vi "Log Data_RT.vi"(5 "FPGA VI Reference":T1, 7 "Total Buffer Size":i32, 8 "error in (no error)":errorcluster, 10 "Acquisition and Logging Configuration":T2={"Data Rate"=1, "Samples per Read"=0, "Number of Reads to Save"=0, "Data File Name"="", "TDMS Properties"=[], "Number of Channels"=4, "Channel Scale Array"=[0.0, 0.0, 0.0, 0.0, 1.0, 1.0, 1.0, 1.0], "Channel Names"=[], "Trigger - RMS Value"=0.0, "Trigger - Channel"=0, "Trigger - Time (Minute)"=0} {"Data Rate" items=["51.200 kS/s (NI 9234)"=1, "25.600 kS/s (NI 9234)"=2, "17.067 kS/s (NI 9234)"=3, "12.800 kS/s (NI 9234)"=4, "10.240 kS/s (NI 9234)"=5, "8.533 kS/s (NI 9234)"=6, "7.314 kS/s (NI 9234)"=7, "6.400 kS/s (NI 9234)"=8, "5.689 kS/s (NI 9234)"=9, "5.120 kS/s (NI 9234)"=10, "4.654 kS/s (NI 9234)"=11, "4.267 kS/s (NI 9234)"=12, "3.938 kS/s (NI 9234)"=13, "3.657 kS/s (NI 9234)"=14, "3.413 kS/s (NI 9234)"=15, "3.200 kS/s (NI 9234)"=16, "3.012 kS/s (NI 9234)"=17, "2.845 kS/s (NI 9234)"=18, "2.695 kS/s (NI 9234)"=19, "2.560 kS/s (NI 9234)"=20, "2.438 kS/s (NI 9234)"=21, "2.328 kS/s (NI 9234)"=22, "2.226 kS/s (NI 9234)"=23, "2.133 kS/s (NI 9234)"=24, "2.048 kS/s (NI 9234)"=25, "1.969 kS/s (NI 9234)"=26, "1.896 kS/s (NI 9234)"=27, "1.829 kS/s (NI 9234)"=28, "1.765 kS/s (NI 9234)"=29, "1.707 kS/s (NI 9234)"=30, "1.652 kS/s (NI 9234)"=31]}, 11 "rt fifo":refnum<k33>) -> (0 "error out":errorcluster)   [LabVIEW 2015]
doc: "Reads waveform data from the DMA FIFO."
uses:
  Globals/Global - Monitoring Variables.vi
  <vilib>/LabVIEW Targets/FPGA/cRIO/shared/nicrio_ModuleControls/nicrio_cRIO-9234_DataRatesRing2.ctl
  controls/Acquisition and Logging Configuration.ctl
  controls/FPGA VI Reference.ctl
  controls/TDMS Properties.ctl
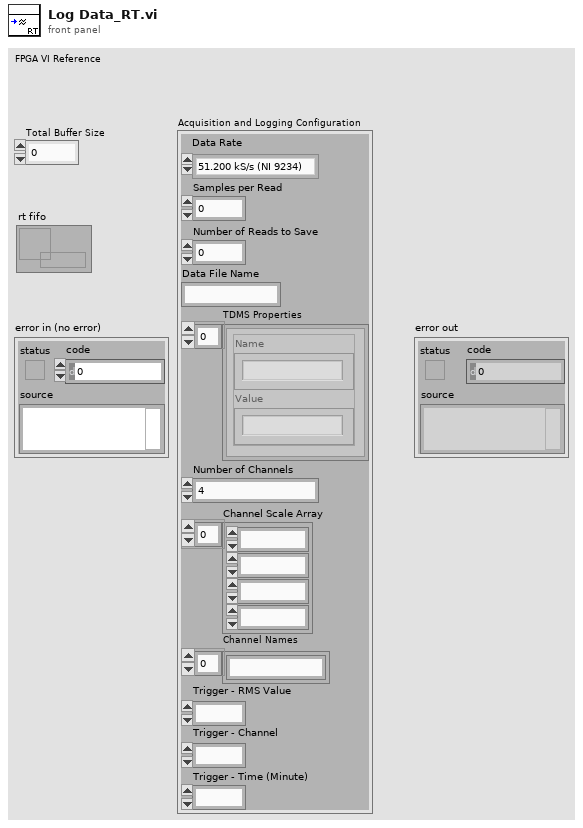
[diagram p1: front panel]
types:
  T1 = typedef "FPGA VI Reference.ctl" = refnum<k20>
  T2 = typedef "Acquisition and Logging Configuration.ctl" = cluster{"Data Rate":T3, "Samples per Read":i32, "Number of Reads to Save":i32, "Data File Name":string, "TDMS Properties":T4[], "Number of Channels":i32, "Channel Scale Array":fxp<+,24,12>[], "Channel Names":string[], "Trigger - RMS Value":dbl, "Trigger - Channel":i32, "Trigger - Time (Minute)":i32}
  T3 = typedef "nicrio_cRIO-9234_DataRatesRing2.ctl" = u8
  T4 = typedef "TDMS Properties.ctl" = cluster{"Name":string, "Value":string}
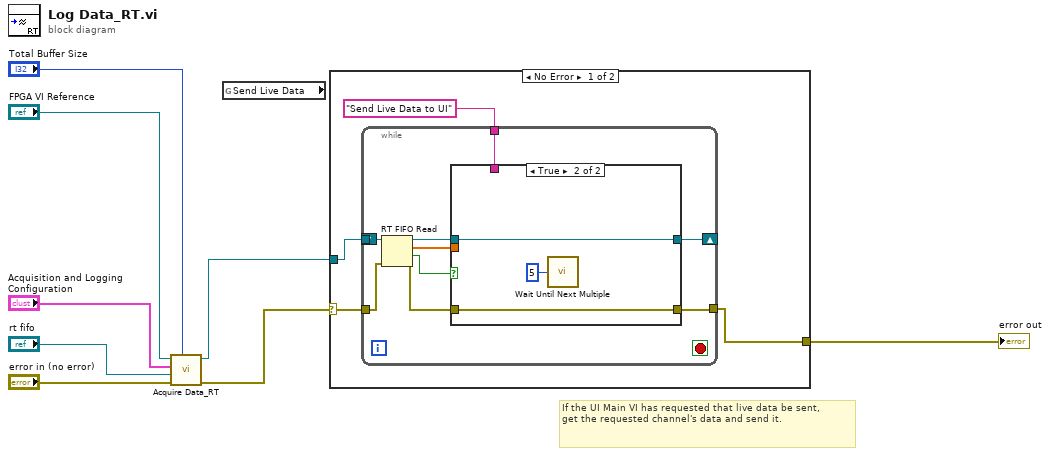
[diagram p0: block diagram]
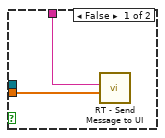
[diagram p2: hidden frame]
diagram:
  # "If the UI Main VI has requested that live data be sent,\nget the requested channel's data and send it."
  n1 = call "Acquire Data_RT.vi"("Total Buffer Size"="Total Buffer Size", "error in (no error)"="error in (no error)", "rt fifo"="rt fifo", "Acquisition and Logging Configuration"="Acquisition and Logging Configuration", "FPGA VI Reference"="FPGA VI Reference") -> ("error out"=w2:errorcluster, "rt fifo out"=w3:refnum<k33>)  [unwired: 4 in, 1 out]
  n2 = global read "Global - Monitoring Variables.vi" "Send Live Data"() -> ()  [unwired: 1 out]
  n3 = case shown="No Error" w2 {
    selector: w2 -> [w10 _]
    tunnel: w3 -> [w12 _]
    tunnel: [w9 _] -> w1
    frame No Error {
      n4 = while {
        tunnel: w12 -> [w21]
        tunnel: "Send Live Data to UI" ("group name in (Untitled)") -> [w19]
        shift-right: [w16] -> _
        shift-left: _ -> [_]
        tunnel: [w15] -> w9
        tunnel: w10 -> [w14]
        stop <- _ stop-if-true
        n5 = RT FIFO Read(0:w21, 3:w14) -> (8:w17:refnum<k33>, 9:w20:sgl[], 10:w18:bool, 11:w13:errorcluster)  [unwired: 2 in, 1 out]
        n6 = case shown="True" w18 {
          tunnel: w20 -> [w23 _]
          tunnel: w19 -> [w22 _]
          tunnel: w17 -> [_ w26]
          tunnel: [_ w26] -> w16
          tunnel: [_ w25] -> w15
          tunnel: w13 -> [_ w25]
          frame False {
            n7 = call "RT - Send Message to UI.vi"("Message Data"=w23, "Message"=w22) -> ()  [unwired: 9 in, 1 out]
          }
          frame True {
            n8 = call "Wait Until Next Multiple"("Count(Ticks)"=u32 5) -> ()  [unwired: 1 out]
          }
        }
      }
    }
    frame Error {
    }
  }
  "error out" <- w1
